vi "Barcode Scanner With Cart and Arm Code.vi"() -> ()   [LabVIEW 2016]
uses:
  <vilib>/NXT/Block Support/NXT_InputPort.ctl
  <vilib>/NXT/Block Support/NXT_OutputPort.ctl
  <vilib>/NXT/Dual Mode Library/Sensors/Touch_Count.vi
  <vilib>/NXT/NXTIO Xnodes/NXTIONodeSubVIs/NXTMotorRunDistance.vi
  <vilib>/NXT/Dual Mode Library/Sensors/EV3_Color_Reflect.vi
  <vilib>/NXT/NXTIO Xnodes/NXTIONodeSubVIs/NXTStopMotors.vi
  <vilib>/NXT/NXTIO Xnodes/NXTIONodeSubVIs/LEGOMoveAllMotorsDistance.vi
  <vilib>/NXT/NXTIO Xnodes/AddressXNode/NXTIOAddress.xnode
  <vilib>/NXT/NXTIO Xnodes/NXTIOXNode/NXTIO.xnode
  <vilib>/NXT/Subs/LVHSConnector.ctl
  <vilib>/NXT/LegoClasses/BrickReference/BrickReference.lvclass
panel:
  out "Marble Type 5":string
  out "Type 1 count 4":string
  out "Type 2 Count 4":string
  out "Marble Type 4 Code":i32[](array[numeric])
  out "Marble Count 4 Code":i32[](array[numeric])
  out "Marble Type 4":string
  out "Type 1 Count 3":string
  out "Type 2 Count 3":string
  out "Marble Count 3":i32[](array[numeric])
  out "Marble Type 3":i32[](array[numeric])
  out "Marble Type 2":string
  out "Type 1 Count 2":string
  out "Type 2 Count 2":string
  out "Marble Count 2 Code":i32[](array[numeric])
  out "Marble Type 2 Code":i32[](array[numeric])
  out "Marble Type code":i32[](array[numeric])
  out "Marble Size code":i32[](array[numeric])
  out "Marble Type":string
  out "Type 2 Count":string
  out "Type 1 Count":string
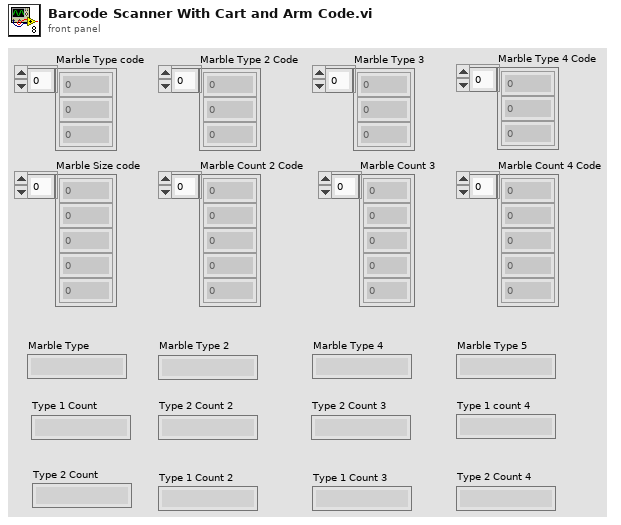
[diagram p1: front panel]
types:
  T1 = typedef "NXT_InputPort.ctl" = u32
  T2 = typedef "LVHSConnector.ctl" = refnum<class "BrickReference.lvclass">
  T3 = typedef "NXT_OutputPort.ctl" = u8
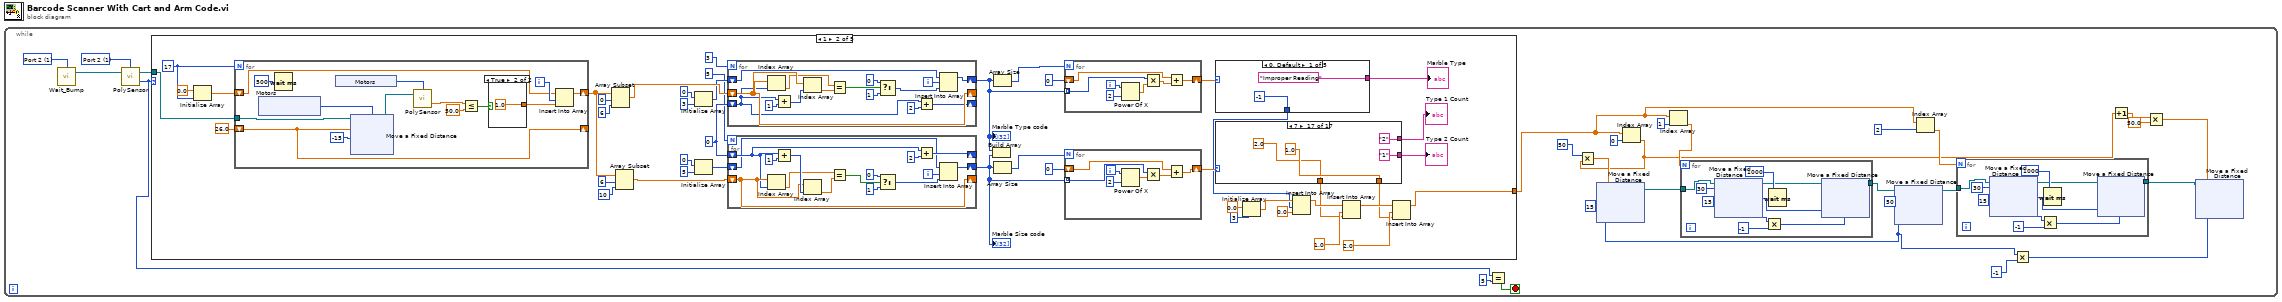
[diagram p0: block diagram]
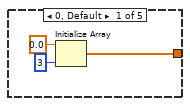
[diagram p2: hidden frame]
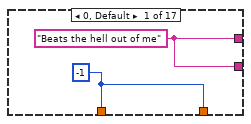
[diagram p3: hidden frame]
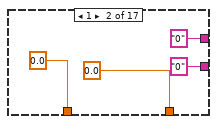
[diagram p4: hidden frame]
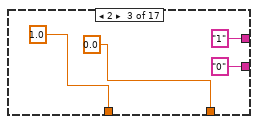
[diagram p5: hidden frame]
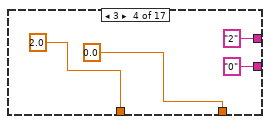
[diagram p6: hidden frame]
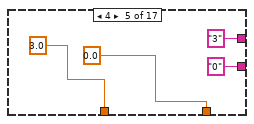
[diagram p7: hidden frame]
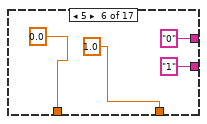
[diagram p8: hidden frame]
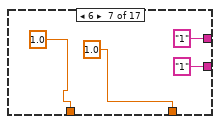
[diagram p9: hidden frame]
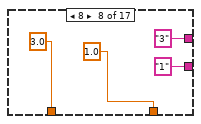
[diagram p10: hidden frame]
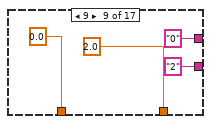
[diagram p11: hidden frame]
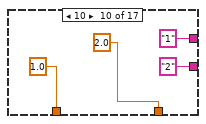
[diagram p12: hidden frame]
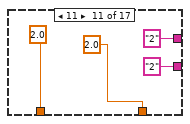
[diagram p13: hidden frame]
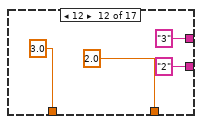
[diagram p14: hidden frame]
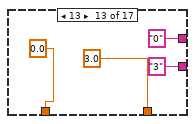
[diagram p15: hidden frame]
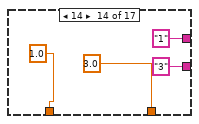
[diagram p16: hidden frame]
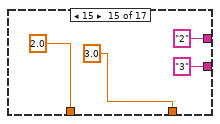
[diagram p17: hidden frame]
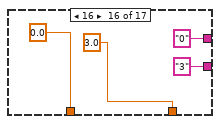
[diagram p18: hidden frame]
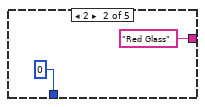
[diagram p19: hidden frame]
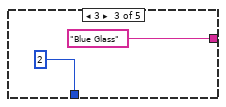
[diagram p20: hidden frame]
diagram:
  n1 = while {
    stop <- w22 stop-if-true
    w7 = i8 15 ("Speed 1")
    w24 = T1 1 items=["Port 1", "Port 2", "Port 3", "Port 4"] ("Port (Port 1)")
    w25 = T1 1 items=["Port 1", "Port 2", "Port 3", "Port 4"] ("Port (Port 1)")
    n2 = call <vilib>:"Wait_Bump.vi"("Port (Port 1)"=w25) -> ("NXT/EV3"=w27:T2)  [unwired: 3 in]
    n3 = call-poly <vilib>:"PolySensor.vi"("NXT/EV3"=w27, "Port (Port 1)"=w24) -> ("Count"=w21:i16, "NXT/EV3"=w26:T2)  [unwired: 1 in]
    n4 = case shown="1" w21 {
      tunnel: w26 -> [_ w108 w305 w497 w696]
      tunnel: [w93 w96 w288 w480 w679] -> w11
      frame 0, Default {
        n5 = Initialize Array(0.0 ("element"), 3 ("dimension size")) -> (w93:dbl[])
      }
      frame 1 {
        w122 = 0
        w139 = 17
        n6 = Initialize Array(0.0, w139) -> (w137:dbl[])
        n7 = for {
          N: w139 -> [_]
          shift-right: [w268] -> w114
          shift-left: w137 -> [w272]
          shift-right: [w265] -> _
          shift-left: 26.0 -> [w265]
          tunnel: w108 -> [w260]
          i -> [w273]
          n8 = xnode "Motors"() -> ("Motor"=w263:T3)
          n9 = Wait (ms)(milliseconds to wait=500) -> ()  [unwired: 1 out]
          n10 = xnode "Motors"() -> ("Sensor"=w267:T1)
          n11 = xnode "Move a Fixed Distance"("Speed 1"=i8 -15, "Distance 1"=w265, "Motors"=w263, "NXT/EV3"=w260) -> ("NXT/EV3"=w264:T2)
          n12 = call-poly <vilib>:"PolySensor.vi"("NXT/EV3"=w264, "Port (Port 1)"=w267) -> ("Scaled Value"=w266:sgl)  [unwired: 1 in, 1 out]
          n13 = Less Or Equal?(x=w266, y=50.0) -> (x <= y?=w270:bool)
          n14 = case shown="True" w270 {
            tunnel: [0.0 1.0] -> w269
            frame False {
            }
            frame True {
            }
          }
          n15 = Insert Into Array(array=w272, index=w273, new element=w269) -> (w268:dbl[])
        }
        n16 = Array Subset(array=w114, index=0, length=6) -> (w130:dbl[])
        n17 = Array Subset(array=w114, index=6, length=10) -> (w126:dbl[])
        n18 = Initialize Array(0, 3 ("dimension size")) -> (w128:i32[])
        n19 = Initialize Array(0, 5 ("dimension size")) -> (w123:i32[])
        n20 = for {
          N: 3 -> [_]
          shift-right: [w257] -> _
          shift-left: w130 -> [w257]
          shift-right: [w249] -> _
          shift-left: w122 -> [w250]
          shift-right: [w247] -> w113
          shift-left: w128 -> [w246]
          i -> [w245]
          n21 = Index Array(array=w257, index=w250) -> (element=w254:dbl)
          n22 = Add(x=w250, y=1) -> (x+y=w258:i32)
          n23 = Index Array(array=w257, index=w258) -> (element=w253:dbl)
          n24 = Equal?(x=w254, y=w253) -> (x = y?=w252:bool)
          n25 = Select(t=0, s=w252, f=1) -> (s? t:f=w251:i32)
          n26 = Add(x=w250, y=2) -> (x+y=w249:i32)
          n27 = Insert Into Array(array=w246, index=w245, new element=w251) -> (w247:i32[])
        }
        "Marble Type code" <- w113
        n28 = for {
          N: 5 -> [_]
          shift-right: [w242] -> _
          shift-left: w126 -> [w242]
          shift-right: [w234] -> _
          shift-left: w122 -> [w235]
          shift-right: [w232] -> w112
          shift-left: w123 -> [w231]
          i -> [w230]
          n29 = Index Array(array=w242, index=w235) -> (element=w239:dbl)
          n30 = Add(x=w235, y=1) -> (x+y=w243:i32)
          n31 = Index Array(array=w242, index=w243) -> (element=w238:dbl)
          n32 = Equal?(x=w239, y=w238) -> (x = y?=w237:bool)
          n33 = Select(t=0, s=w237, f=1) -> (s? t:f=w236:i32)
          n34 = Add(x=w235, y=2) -> (x+y=w234:i32)
          n35 = Insert Into Array(array=w231, index=w230, new element=w236) -> (w232:i32[])
        }
        "Marble Size code" <- w112
        n36 = Build Array(w113, w112) -> ()  [unwired: 1 out]
        n37 = Array Size(array=w113) -> (size(s)=w120:i32)
        n38 = Array Size(array=w112) -> (size(s)=w117:i32)
        n39 = for {
          N: w120 -> [_]
          tunnel: w113 -> [w150] mode=indexing
          shift-right: [w147] -> w118
          shift-left: 0 -> [w148]
          i -> [w152]
          n40 = Power Of X(1:2, 2:w152) -> (0:w151:dbl)
          n41 = Multiply(x=w150, y=w151) -> (x*y=w149:dbl)
          n42 = Add(x=w148, y=w149) -> (x+y=w147:dbl)
        }
        n43 = for {
          N: w117 -> [_]
          tunnel: w112 -> [w143] mode=indexing
          shift-right: [w140] -> w115
          shift-left: 0 -> [w141]
          i -> [w145]
          n44 = Power Of X(1:2, 2:w145) -> (0:w144:dbl)
          n45 = Multiply(x=w143, y=w144) -> (x*y=w142:dbl)
          n46 = Add(x=w141, y=w142) -> (x+y=w140:dbl)
        }
        n47 = case shown="0, Default" w118 {
          tunnel: ["Improper Reading" "Red Glass" "Blue Glass" "White Glass" "Steel/HDPE"] -> w109
          tunnel: [-1 0 2 4 6] -> w99
          frame 0, Default {
          }
          frame 2 {
          }
          frame 3 {
          }
          frame 1 {
          }
          frame 4 {
          }
        }
        "Marble Type" <- w109
        n48 = case shown="7" w115 {
          tunnel: [w155 "0" "1" "2" "3" "0" "1" "3" "0" "1" "2" "3" "0" "1" "2" "0" "2"] -> w111
          tunnel: [w155 "0" "0" "0" "0" "1" "1" "1" "2" "2" "2" "2" "3" "3" "3" "3" "1"] -> w110
          tunnel: [w154 0.0 ("new element/subarray") 1.0 ("new element/subarray") 2.0 ("new element/subarray") 3.0 ("new element/subarray") 0.0 ("new element/subarray") 1.0 ("new element/subarray") 3.0 ("new element/subarray") 0.0 ("new element/subarray") 1.0 ("new element/subarray") 2.0 ("new element/subarray") 3.0 ("new element/subarray") 0.0 ("new element/subarray") 1.0 ("new element/subarray") 2.0 ("new element/subarray") 0.0 ("new element/subarray") 2.0 ("new element/subarray")] -> w98
          tunnel: [w154 0.0 ("new element/subarray") 0.0 ("new element/subarray") 0.0 ("new element/subarray") 0.0 ("new element/subarray") 1.0 ("new element/subarray") 1.0 ("new element/subarray") 1.0 ("new element/subarray") 2.0 ("new element/subarray") 2.0 ("new element/subarray") 2.0 ("new element/subarray") 2.0 ("new element/subarray") 3.0 ("new element/subarray") 3.0 ("new element/subarray") 3.0 ("new element/subarray") 3.0 ("new element/subarray") 1.0 ("new element/subarray")] -> w97
          frame 0, Default {
            w154 = -1
            w155 = "Beats the hell out of me"
          }
          frame 1 {
          }
          frame 2 {
          }
          frame 3 {
          }
          frame 4 {
          }
          frame 5 {
          }
          frame 6 {
          }
          frame 8 {
          }
          frame 9 {
          }
          frame 10 {
          }
          frame 11 {
          }
          frame 12 {
          }
          frame 13 {
          }
          frame 14 {
          }
          frame 15 {
          }
          frame 16 {
          }
          frame 7 {
          }
        }
        "Type 2 Count" <- w110
        "Type 1 Count" <- w111
        n49 = Initialize Array(0.0 ("element"), 3 ("dimension size")) -> (w105:dbl[])
        n50 = Insert Into Array(array=w105, index=w99, new element=0.0 ("new element/subarray")) -> (w104:dbl[])
        n51 = Insert Into Array(array=w104, index=1.0 ("new element/subarray"), new element=w98) -> (w103:dbl[])
        n52 = Insert Into Array(array=w103, index=2.0 ("new element/subarray"), new element=w97) -> (w96:dbl[])
      }
      frame 2 {
        w314 = 0
        w331 = 17
        n53 = Initialize Array(0.0, w331) -> (w329:dbl[])
        n54 = for {
          N: w331 -> [_]
          shift-right: [w460] -> w308
          shift-left: w329 -> [w464]
          shift-right: [w457] -> _
          shift-left: 26.0 -> [w457]
          tunnel: w305 -> [w452]
          i -> [w465]
          n55 = xnode "Motors"() -> ("Motor"=w455:T3)
          n56 = Wait (ms)(milliseconds to wait=500) -> ()  [unwired: 1 out]
          n57 = xnode "Motors"() -> ("Sensor"=w459:T1)
          n58 = xnode "Move a Fixed Distance"("Speed 1"=i8 -15, "Distance 1"=w457, "Motors"=w455, "NXT/EV3"=w452) -> ("NXT/EV3"=w456:T2)
          n59 = call-poly <vilib>:"PolySensor.vi"("NXT/EV3"=w456, "Port (Port 1)"=w459) -> ("Scaled Value"=w458:sgl)  [unwired: 1 in, 1 out]
          n60 = Less Or Equal?(x=w458, y=50.0) -> (x <= y?=w462:bool)
          n61 = case shown="True" w462 {
            tunnel: [0.0 1.0] -> w461
            frame False {
            }
            frame True {
            }
          }
          n62 = Insert Into Array(array=w464, index=w465, new element=w461) -> (w460:dbl[])
        }
        n63 = Array Subset(array=w308, index=0, length=6) -> (w322:dbl[])
        n64 = Array Subset(array=w308, index=6, length=10) -> (w318:dbl[])
        n65 = Initialize Array(0, 3 ("dimension size")) -> (w320:i32[])
        n66 = for {
          N: 3 -> [_]
          shift-right: [w449] -> _
          shift-left: w322 -> [w449]
          shift-right: [w441] -> _
          shift-left: w314 -> [w442]
          shift-right: [w439] -> w307
          shift-left: w320 -> [w438]
          i -> [w437]
          n67 = Index Array(array=w449, index=w442) -> (element=w446:dbl)
          n68 = Add(x=w442, y=1) -> (x+y=w450:i32)
          n69 = Index Array(array=w449, index=w450) -> (element=w445:dbl)
          n70 = Equal?(x=w446, y=w445) -> (x = y?=w444:bool)
          n71 = Select(t=0, s=w444, f=1) -> (s? t:f=w443:i32)
          n72 = Add(x=w442, y=2) -> (x+y=w441:i32)
          n73 = Insert Into Array(array=w438, index=w437, new element=w443) -> (w439:i32[])
        }
        "Marble Type 2 Code" <- w307
        n74 = Initialize Array(0, 5 ("dimension size")) -> (w315:i32[])
        n75 = for {
          N: 5 -> [_]
          shift-right: [w434] -> _
          shift-left: w318 -> [w434]
          shift-right: [w426] -> _
          shift-left: w314 -> [w427]
          shift-right: [w424] -> w306
          shift-left: w315 -> [w423]
          i -> [w422]
          n76 = Index Array(array=w434, index=w427) -> (element=w431:dbl)
          n77 = Add(x=w427, y=1) -> (x+y=w435:i32)
          n78 = Index Array(array=w434, index=w435) -> (element=w430:dbl)
          n79 = Equal?(x=w431, y=w430) -> (x = y?=w429:bool)
          n80 = Select(t=0, s=w429, f=1) -> (s? t:f=w428:i32)
          n81 = Add(x=w427, y=2) -> (x+y=w426:i32)
          n82 = Insert Into Array(array=w423, index=w422, new element=w428) -> (w424:i32[])
        }
        "Marble Count 2 Code" <- w306
        n83 = Array Size(array=w307) -> (size(s)=w312:i32)
        n84 = Array Size(array=w306) -> (size(s)=w310:i32)
        n85 = for {
          N: w312 -> [_]
          tunnel: w307 -> [w418] mode=indexing
          shift-right: [w415] -> w291
          shift-left: 0 -> [w416]
          i -> [w420]
          n86 = Power Of X(1:2, 2:w420) -> (0:w419:dbl)
          n87 = Multiply(x=w418, y=w419) -> (x*y=w417:dbl)
          n88 = Add(x=w416, y=w417) -> (x+y=w415:dbl)
        }
        n89 = for {
          N: w310 -> [_]
          tunnel: w306 -> [w411] mode=indexing
          shift-right: [w408] -> w289
          shift-left: 0 -> [w409]
          i -> [w413]
          n90 = Power Of X(1:2, 2:w413) -> (0:w412:dbl)
          n91 = Multiply(x=w411, y=w412) -> (x*y=w410:dbl)
          n92 = Add(x=w409, y=w410) -> (x+y=w408:dbl)
        }
        n93 = case shown="0, Default" w291 {
          tunnel: ["Improper Reading" "Red Glass" "Blue Glass" "White Glass" "Steel/HDPE"] -> w292
          tunnel: [-1 0 2 4 6] -> w290
          frame 0, Default {
          }
          frame 2 {
          }
          frame 3 {
          }
          frame 1 {
          }
          frame 4 {
          }
        }
        "Marble Type 2" <- w292
        n94 = case shown="7" w289 {
          tunnel: [w333 "0" "1" "2" "3" "0" "1" "3" "0" "1" "2" "3" "0" "1" "2" "0" "2"] -> w294
          tunnel: [w333 "0" "0" "0" "0" "1" "1" "1" "2" "2" "2" "2" "3" "3" "3" "3" "1"] -> w293
          tunnel: [w332 0.0 ("new element/subarray") 1.0 ("new element/subarray") 2.0 ("new element/subarray") 3.0 ("new element/subarray") 0.0 ("new element/subarray") 1.0 ("new element/subarray") 3.0 ("new element/subarray") 0.0 ("new element/subarray") 1.0 ("new element/subarray") 2.0 ("new element/subarray") 3.0 ("new element/subarray") 0.0 ("new element/subarray") 1.0 ("new element/subarray") 2.0 ("new element/subarray") 0.0 ("new element/subarray") 2.0 ("new element/subarray")] -> w296
          tunnel: [w332 0.0 ("new element/subarray") 0.0 ("new element/subarray") 0.0 ("new element/subarray") 0.0 ("new element/subarray") 1.0 ("new element/subarray") 1.0 ("new element/subarray") 1.0 ("new element/subarray") 2.0 ("new element/subarray") 2.0 ("new element/subarray") 2.0 ("new element/subarray") 2.0 ("new element/subarray") 3.0 ("new element/subarray") 3.0 ("new element/subarray") 3.0 ("new element/subarray") 3.0 ("new element/subarray") 1.0 ("new element/subarray")] -> w295
          frame 0, Default {
            w332 = -1
            w333 = "Beats the hell out of me"
          }
          frame 1 {
          }
          frame 2 {
          }
          frame 3 {
          }
          frame 4 {
          }
          frame 5 {
          }
          frame 6 {
          }
          frame 8 {
          }
          frame 9 {
          }
          frame 10 {
          }
          frame 11 {
          }
          frame 12 {
          }
          frame 13 {
          }
          frame 14 {
          }
          frame 15 {
          }
          frame 16 {
          }
          frame 7 {
          }
        }
        "Type 1 Count 2" <- w294
        "Type 2 Count 2" <- w293
        n95 = Initialize Array(0.0 ("element"), 3 ("dimension size")) -> (w302:dbl[])
        n96 = Insert Into Array(array=w302, index=w290, new element=0.0 ("new element/subarray")) -> (w301:dbl[])
        n97 = Insert Into Array(array=w301, index=1.0 ("new element/subarray"), new element=w296) -> (w300:dbl[])
        n98 = Insert Into Array(array=w300, index=2.0 ("new element/subarray"), new element=w295) -> (w288:dbl[])
      }
      frame 3 {
        w516 = 0
        w499 = 17
        n99 = Initialize Array(0.0, w499) -> (w501:dbl[])
        n100 = for {
          N: w499 -> [_]
          shift-right: [w653] -> w522
          shift-left: w501 -> [w657]
          shift-right: [w650] -> _
          shift-left: 26.0 -> [w650]
          tunnel: w497 -> [w644]
          i -> [w658]
          n101 = xnode "Motors"() -> ("Motor"=w645:T3)
          n102 = xnode "Motors"() -> ("Motor"=w648:T3)
          n103 = Wait (ms)(milliseconds to wait=500) -> ()  [unwired: 1 out]
          n104 = xnode "Stop Motors"("Motors"=w645) -> ()  [unwired: 1 in, 1 out]
          n105 = xnode "Motors"() -> ("Sensor"=w652:T1)
          n106 = xnode "Move a Fixed Distance"("Speed 1"=i8 -15, "Distance 1"=w650, "Motors"=w648, "NXT/EV3"=w644) -> ("NXT/EV3"=w649:T2)
          n107 = call-poly <vilib>:"PolySensor.vi"("NXT/EV3"=w649, "Port (Port 1)"=w652) -> ("Scaled Value"=w651:sgl)  [unwired: 1 in, 1 out]
          n108 = Less Or Equal?(x=w651, y=50.0) -> (x <= y?=w655:bool)
          n109 = case shown="True" w655 {
            tunnel: [0.0 1.0] -> w654
            frame False {
            }
            frame True {
            }
          }
          n110 = Insert Into Array(array=w657, index=w658, new element=w654) -> (w653:dbl[])
        }
        n111 = Array Subset(array=w522, index=0, length=6) -> (w508:dbl[])
        n112 = Array Subset(array=w522, index=6, length=10) -> (w512:dbl[])
        n113 = Initialize Array(0, 3 ("dimension size")) -> (w510:i32[])
        n114 = for {
          N: 3 -> [_]
          shift-right: [w641] -> _
          shift-left: w508 -> [w641]
          shift-right: [w633] -> _
          shift-left: w516 -> [w634]
          shift-right: [w631] -> w523
          shift-left: w510 -> [w630]
          i -> [w629]
          n115 = Index Array(array=w641, index=w634) -> (element=w638:dbl)
          n116 = Add(x=w634, y=1) -> (x+y=w642:i32)
          n117 = Index Array(array=w641, index=w642) -> (element=w637:dbl)
          n118 = Equal?(x=w638, y=w637) -> (x = y?=w636:bool)
          n119 = Select(t=0, s=w636, f=1) -> (s? t:f=w635:i32)
          n120 = Add(x=w634, y=2) -> (x+y=w633:i32)
          n121 = Insert Into Array(array=w630, index=w629, new element=w635) -> (w631:i32[])
        }
        "Marble Type 3" <- w523
        n122 = Initialize Array(0, 5 ("dimension size")) -> (w515:i32[])
        n123 = for {
          N: 5 -> [_]
          shift-right: [w626] -> _
          shift-left: w512 -> [w626]
          shift-right: [w618] -> _
          shift-left: w516 -> [w619]
          shift-right: [w616] -> w498
          shift-left: w515 -> [w615]
          i -> [w614]
          n124 = Index Array(array=w626, index=w619) -> (element=w623:dbl)
          n125 = Add(x=w619, y=1) -> (x+y=w627:i32)
          n126 = Index Array(array=w626, index=w627) -> (element=w622:dbl)
          n127 = Equal?(x=w623, y=w622) -> (x = y?=w621:bool)
          n128 = Select(t=0, s=w621, f=1) -> (s? t:f=w620:i32)
          n129 = Add(x=w619, y=2) -> (x+y=w618:i32)
          n130 = Insert Into Array(array=w615, index=w614, new element=w620) -> (w616:i32[])
        }
        "Marble Count 3" <- w498
        n131 = Array Size(array=w523) -> (size(s)=w518:i32)
        n132 = Array Size(array=w498) -> (size(s)=w520:i32)
        n133 = for {
          N: w518 -> [_]
          tunnel: w523 -> [w610] mode=indexing
          shift-right: [w607] -> w481
          shift-left: 0 -> [w608]
          i -> [w612]
          n134 = Power Of X(1:2, 2:w612) -> (0:w611:dbl)
          n135 = Multiply(x=w610, y=w611) -> (x*y=w609:dbl)
          n136 = Add(x=w608, y=w609) -> (x+y=w607:dbl)
        }
        n137 = for {
          N: w520 -> [_]
          tunnel: w498 -> [w603] mode=indexing
          shift-right: [w600] -> w482
          shift-left: 0 -> [w601]
          i -> [w605]
          n138 = Power Of X(1:2, 2:w605) -> (0:w604:dbl)
          n139 = Multiply(x=w603, y=w604) -> (x*y=w602:dbl)
          n140 = Add(x=w601, y=w602) -> (x+y=w600:dbl)
        }
        n141 = case shown="0, Default" w481 {
          tunnel: ["Improper Reading" "Red Glass" "Blue Glass" "White Glass" "Steel/HDPE"] -> w486
          tunnel: [-1 0 2 4 6] -> w483
          frame 0, Default {
          }
          frame 2 {
          }
          frame 3 {
          }
          frame 1 {
          }
          frame 4 {
          }
        }
        "Marble Type 4" <- w486
        n142 = case shown="7" w482 {
          tunnel: [w525 "0" "1" "2" "3" "0" "1" "3" "0" "1" "2" "3" "0" "1" "2" "0" "2"] -> w485
          tunnel: [w525 "0" "0" "0" "0" "1" "1" "1" "2" "2" "2" "2" "3" "3" "3" "3" "1"] -> w484
          tunnel: [w524 0.0 ("new element/subarray") 1.0 ("new element/subarray") 2.0 ("new element/subarray") 3.0 ("new element/subarray") 0.0 ("new element/subarray") 1.0 ("new element/subarray") 3.0 ("new element/subarray") 0.0 ("new element/subarray") 1.0 ("new element/subarray") 2.0 ("new element/subarray") 3.0 ("new element/subarray") 0.0 ("new element/subarray") 1.0 ("new element/subarray") 2.0 ("new element/subarray") 0.0 ("new element/subarray") 2.0 ("new element/subarray")] -> w488
          tunnel: [w524 0.0 ("new element/subarray") 0.0 ("new element/subarray") 0.0 ("new element/subarray") 0.0 ("new element/subarray") 1.0 ("new element/subarray") 1.0 ("new element/subarray") 1.0 ("new element/subarray") 2.0 ("new element/subarray") 2.0 ("new element/subarray") 2.0 ("new element/subarray") 2.0 ("new element/subarray") 3.0 ("new element/subarray") 3.0 ("new element/subarray") 3.0 ("new element/subarray") 3.0 ("new element/subarray") 1.0 ("new element/subarray")] -> w487
          frame 0, Default {
            w524 = -1
            w525 = "Beats the hell out of me"
          }
          frame 1 {
          }
          frame 2 {
          }
          frame 3 {
          }
          frame 4 {
          }
          frame 5 {
          }
          frame 6 {
          }
          frame 8 {
          }
          frame 9 {
          }
          frame 10 {
          }
          frame 11 {
          }
          frame 12 {
          }
          frame 13 {
          }
          frame 14 {
          }
          frame 15 {
          }
          frame 16 {
          }
          frame 7 {
          }
        }
        "Type 1 Count 3" <- w485
        "Type 2 Count 3" <- w484
        n143 = Initialize Array(0.0 ("element"), 3 ("dimension size")) -> (w494:dbl[])
        n144 = Insert Into Array(array=w494, index=w483, new element=0.0 ("new element/subarray")) -> (w493:dbl[])
        n145 = Insert Into Array(array=w493, index=1.0 ("new element/subarray"), new element=w488) -> (w492:dbl[])
        n146 = Insert Into Array(array=w492, index=2.0 ("new element/subarray"), new element=w487) -> (w480:dbl[])
      }
      frame 4 {
        w714 = 0
        w697 = 17
        n147 = Initialize Array(0.0, w697) -> (w699:dbl[])
        n148 = for {
          N: w697 -> [_]
          shift-right: [w854] -> w720
          shift-left: w699 -> [w858]
          shift-right: [w851] -> _
          shift-left: 26.0 -> [w851]
          tunnel: w696 -> [w845]
          tunnel: [w843] -> _
          i -> [w859]
          n149 = xnode "Motors"() -> ("Motor"=w849:T3)
          n150 = Wait (ms)(milliseconds to wait=500) -> ()  [unwired: 1 out]
          n151 = xnode "Motors"() -> ("Sensor"=w853:T1)
          n152 = xnode "Move a Fixed Distance"("Speed 1"=i8 -15, "Distance 1"=w851, "Motors"=w849, "NXT/EV3"=w845) -> ("NXT/EV3"=w850:T2)
          n153 = xnode "Motors"() -> ("Motor"=w846:T3)
          n154 = call-poly <vilib>:"PolySensor.vi"("NXT/EV3"=w850, "Port (Port 1)"=w853) -> ("Scaled Value"=w852:sgl, "NXT/EV3"=w844:T2)  [unwired: 1 in]
          n155 = xnode "Stop Motors"("Motors"=w846, "NXT/EV3"=w844) -> ("NXT/EV3"=w843:T2)
          n156 = Less Or Equal?(x=w852, y=50.0) -> (x <= y?=w856:bool)
          n157 = case shown="True" w856 {
            tunnel: [0.0 1.0] -> w855
            frame False {
            }
            frame True {
            }
          }
          n158 = Insert Into Array(array=w858, index=w859, new element=w855) -> (w854:dbl[])
        }
        n159 = Array Subset(array=w720, index=0, length=6) -> (w706:dbl[])
        n160 = Array Subset(array=w720, index=6, length=10) -> (w710:dbl[])
        n161 = Initialize Array(0, 3 ("dimension size")) -> (w708:i32[])
        n162 = for {
          N: 3 -> [_]
          shift-right: [w840] -> _
          shift-left: w706 -> [w840]
          shift-right: [w832] -> _
          shift-left: w714 -> [w833]
          shift-right: [w830] -> w721
          shift-left: w708 -> [w829]
          i -> [w828]
          n163 = Index Array(array=w840, index=w833) -> (element=w837:dbl)
          n164 = Add(x=w833, y=1) -> (x+y=w841:i32)
          n165 = Index Array(array=w840, index=w841) -> (element=w836:dbl)
          n166 = Equal?(x=w837, y=w836) -> (x = y?=w835:bool)
          n167 = Select(t=0, s=w835, f=1) -> (s? t:f=w834:i32)
          n168 = Add(x=w833, y=2) -> (x+y=w832:i32)
          n169 = Insert Into Array(array=w829, index=w828, new element=w834) -> (w830:i32[])
        }
        "Marble Type 4 Code" <- w721
        n170 = Initialize Array(0, 5 ("dimension size")) -> (w713:i32[])
        n171 = for {
          N: 5 -> [_]
          shift-right: [w825] -> _
          shift-left: w710 -> [w825]
          shift-right: [w817] -> _
          shift-left: w714 -> [w818]
          shift-right: [w815] -> w722
          shift-left: w713 -> [w814]
          i -> [w813]
          n172 = Index Array(array=w825, index=w818) -> (element=w822:dbl)
          n173 = Add(x=w818, y=1) -> (x+y=w826:i32)
          n174 = Index Array(array=w825, index=w826) -> (element=w821:dbl)
          n175 = Equal?(x=w822, y=w821) -> (x = y?=w820:bool)
          n176 = Select(t=0, s=w820, f=1) -> (s? t:f=w819:i32)
          n177 = Add(x=w818, y=2) -> (x+y=w817:i32)
          n178 = Insert Into Array(array=w814, index=w813, new element=w819) -> (w815:i32[])
        }
        "Marble Count 4 Code" <- w722
        n179 = Array Size(array=w721) -> (size(s)=w716:i32)
        n180 = Array Size(array=w722) -> (size(s)=w718:i32)
        n181 = for {
          N: w716 -> [_]
          tunnel: w721 -> [w809] mode=indexing
          shift-right: [w806] -> w680
          shift-left: 0 -> [w807]
          i -> [w811]
          n182 = Power Of X(1:2, 2:w811) -> (0:w810:dbl)
          n183 = Multiply(x=w809, y=w810) -> (x*y=w808:dbl)
          n184 = Add(x=w807, y=w808) -> (x+y=w806:dbl)
        }
        n185 = for {
          N: w718 -> [_]
          tunnel: w722 -> [w802] mode=indexing
          shift-right: [w799] -> w681
          shift-left: 0 -> [w800]
          i -> [w804]
          n186 = Power Of X(1:2, 2:w804) -> (0:w803:dbl)
          n187 = Multiply(x=w802, y=w803) -> (x*y=w801:dbl)
          n188 = Add(x=w800, y=w801) -> (x+y=w799:dbl)
        }
        n189 = case shown="0, Default" w680 {
          tunnel: ["Improper Reading" "Red Glass" "Blue Glass" "White Glass" "Steel/HDPE"] -> w685
          tunnel: [-1 0 2 4 6] -> w682
          frame 0, Default {
          }
          frame 2 {
          }
          frame 3 {
          }
          frame 1 {
          }
          frame 4 {
          }
        }
        "Marble Type 5" <- w685
        n190 = case shown="7" w681 {
          tunnel: [w724 "0" "1" "2" "3" "0" "1" "3" "0" "1" "2" "3" "0" "1" "2" "0" "2"] -> w684
          tunnel: [w724 "0" "0" "0" "0" "1" "1" "1" "2" "2" "2" "2" "3" "3" "3" "3" "1"] -> w683
          tunnel: [w723 0.0 ("new element/subarray") 1.0 ("new element/subarray") 2.0 ("new element/subarray") 3.0 ("new element/subarray") 0.0 ("new element/subarray") 1.0 ("new element/subarray") 3.0 ("new element/subarray") 0.0 ("new element/subarray") 1.0 ("new element/subarray") 2.0 ("new element/subarray") 3.0 ("new element/subarray") 0.0 ("new element/subarray") 1.0 ("new element/subarray") 2.0 ("new element/subarray") 0.0 ("new element/subarray") 2.0 ("new element/subarray")] -> w687
          tunnel: [w723 0.0 ("new element/subarray") 0.0 ("new element/subarray") 0.0 ("new element/subarray") 0.0 ("new element/subarray") 1.0 ("new element/subarray") 1.0 ("new element/subarray") 1.0 ("new element/subarray") 2.0 ("new element/subarray") 2.0 ("new element/subarray") 2.0 ("new element/subarray") 2.0 ("new element/subarray") 3.0 ("new element/subarray") 3.0 ("new element/subarray") 3.0 ("new element/subarray") 3.0 ("new element/subarray") 1.0 ("new element/subarray")] -> w686
          frame 0, Default {
            w723 = -1
            w724 = "Beats the hell out of me"
          }
          frame 1 {
          }
          frame 2 {
          }
          frame 3 {
          }
          frame 4 {
          }
          frame 5 {
          }
          frame 6 {
          }
          frame 8 {
          }
          frame 9 {
          }
          frame 10 {
          }
          frame 11 {
          }
          frame 12 {
          }
          frame 13 {
          }
          frame 14 {
          }
          frame 15 {
          }
          frame 16 {
          }
          frame 7 {
          }
        }
        "Type 1 count 4" <- w684
        "Type 2 Count 4" <- w683
        n191 = Initialize Array(0.0 ("element"), 3 ("dimension size")) -> (w693:dbl[])
        n192 = Insert Into Array(array=w693, index=w682, new element=0.0 ("new element/subarray")) -> (w692:dbl[])
        n193 = Insert Into Array(array=w692, index=1.0 ("new element/subarray"), new element=w687) -> (w691:dbl[])
        n194 = Insert Into Array(array=w691, index=2.0 ("new element/subarray"), new element=w686) -> (w679:dbl[])
      }
    }
    n195 = Equal?(x=w21, y=5) -> (x = y?=w22:bool)
    n196 = Index Array(array=w11, index=0) -> (element=w5:dbl)
    n197 = Multiply(x=50, y=w5) -> (x*y=w18:dbl)
    n198 = xnode "Move a Fixed Distance"("Speed 1"=w7, "Distance 1"=w18) -> ("NXT/EV3"=w17:T2)  [unwired: 2 in]
    n199 = Index Array(array=w11, index=1) -> (element=w15:dbl)
    n200 = for {
      N: w15 -> [_]
      tunnel: w17 -> [w71]
      tunnel: [w64] -> w14
      w69 = 30 ("Distance 1")
      w67 = i8 15 ("Speed 1")
      n201 = xnode "Move a Fixed Distance"("Speed 1"=w67, "Distance 1"=w69, "NXT/EV3"=w71) -> ("NXT/EV3"=w65:T2)  [unwired: 1 in]
      n202 = Multiply(x=w67, y=-1) -> (x*y=w66:i32)
      n203 = Wait (ms)(milliseconds to wait=u32 1000) -> ()  [unwired: 1 out]
      n204 = xnode "Move a Fixed Distance"("Speed 1"=w66, "Distance 1"=w69, "NXT/EV3"=w65) -> ("NXT/EV3"=w64:T2)  [unwired: 1 in]
    }
    n205 = xnode "Move a Fixed Distance"("Speed 1"=w7, "Distance 1"=50, "NXT/EV3"=w14) -> ("NXT/EV3"=w13:T2)  [unwired: 1 in]
    n206 = Index Array(array=w11, index=2) -> (element=w9:dbl)
    n207 = for {
      N: w9 -> [_]
      tunnel: w13 -> [w49]
      tunnel: [w42] -> w1
      w47 = 30 ("Distance 1")
      w45 = i8 15 ("Speed 1")
      n208 = xnode "Move a Fixed Distance"("Speed 1"=w45, "Distance 1"=w47, "NXT/EV3"=w49) -> ("NXT/EV3"=w43:T2)  [unwired: 1 in]
      n209 = Multiply(x=w45, y=-1) -> (x*y=w44:i32)
      n210 = Wait (ms)(milliseconds to wait=u32 1000) -> ()  [unwired: 1 out]
      n211 = xnode "Move a Fixed Distance"("Speed 1"=w44, "Distance 1"=w47, "NXT/EV3"=w43) -> ("NXT/EV3"=w42:T2)  [unwired: 1 in]
    }
    n212 = Multiply(x=w7, y=-1) -> (x*y=w6:i32)
    n213 = Increment(x=w5) -> (x+1=w4:dbl)
    n214 = Multiply(x=w4, y=50.0) -> (x*y=w2:dbl)
    n215 = xnode "Move a Fixed Distance"("Speed 1"=w6, "Distance 1"=w2, "NXT/EV3"=w1) -> ()  [unwired: 1 in, 1 out]
  }
